vi "Setup.vi"(8 "error in (no error)":errorcluster caption="Fehler (Eingang, kein Fehler)", 9 "Baudrate":u32=250000, 10 "VISA resource name":refnum<visa-resource-name>, 11 "MoveoSerial Eingang":refnum<class "MoveoSerial.lvclass">) -> (0 "error out":errorcluster caption="Fehler (Ausgang)", 3 "MoveoSerial Ausgang":refnum<class "MoveoSerial.lvclass">)   [LabVIEW 2019, in "MoveoSerial.lvclass"]
uses:
  MoveoSerial.lvclass
  MoveoSerial.lvclass/MoveoSerial.ctl
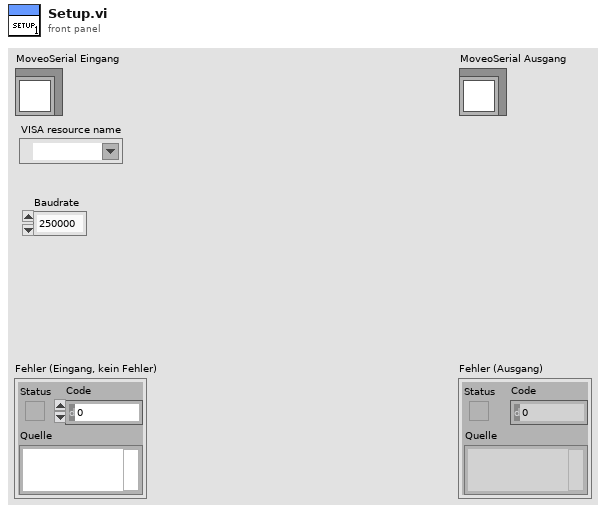
[diagram p1: front panel]
types:
  T1 = typedef "Serial - Settings.ctl" = cluster{"Baudrate":u32, "Datenbits":u16, "Parität":enum16{"None", "Odd", "Even", "Mark", "Space"}, "Stoppbits":u16, "Ablaufsteuerung":u16}
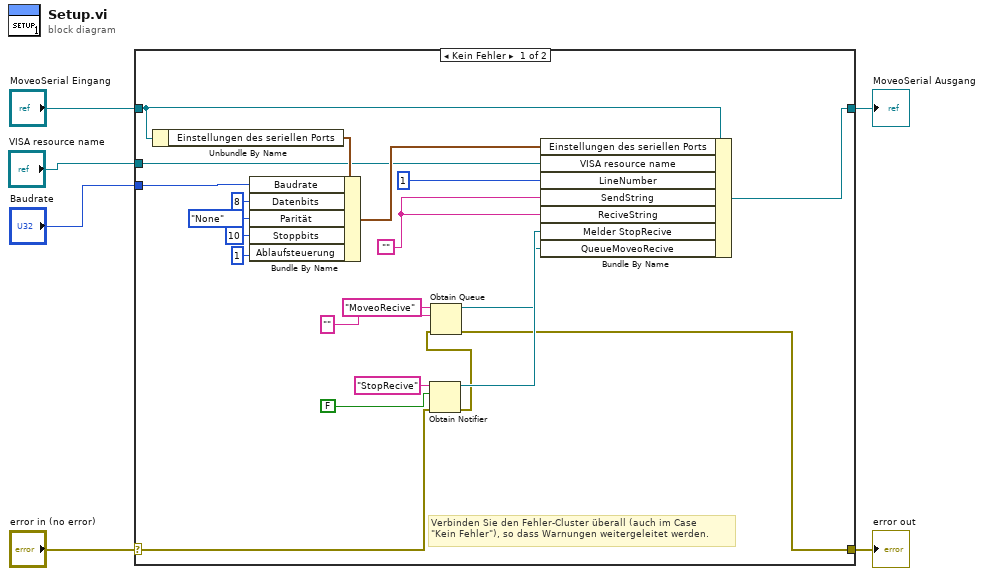
[diagram p0: block diagram]
diagram:
  n1 = case shown="Kein Fehler" "error in (no error)" {
    selector: "error in (no error)" -> [w13 w29]
    tunnel: [w10 w29] -> w5
    tunnel: [w27 w28] -> w3
    tunnel: "MoveoSerial Eingang" -> [w26 w28]
    tunnel: "Baudrate" -> [w19 _]
    tunnel: "VISA resource name" -> [w18 _]
    frame No Error {
      w16 = ""
      # "Verbinden Sie den Fehler-Cluster überall (auch im Case\n\"Kein Fehler\"), so dass Warnungen weitergeleitet werden."
      n2 = Unbundle By Name(w26) -> ("Einstellungen des seriellen Ports"=w25:T1)
      n3 = Bundle By Name(cluster=w25, "Baudrate"=w19, "Datenbits"=u16 8, "Parität"=enum16{"None", "Odd", "Even", "Mark", "Space"}."None", "Stoppbits"=u16 10, "Ablaufsteuerung"=u16 1) -> (w24:T1)
      n4 = Obtain Notifier(name (unnamed)="StopRecive" ("Name (unbenannt)"), notification data type=FALSE, error in (no error)=w13) -> (notifier out=w12:refnum<notifier>, error out=w11:errorcluster)  [unwired: 1 in, 1 out]
      n5 = Obtain Queue(name (unnamed)="MoveoRecive" ("Name (unbenannt)"), element data type="", error in (no error)=w11) -> (queue out=w9:refnum<queue>, error out=w10:errorcluster)  [unwired: 2 in, 1 out]
      n6 = Bundle By Name(cluster=w26, "Einstellungen des seriellen Ports"=w24, "VISA resource name"=w18, "LineNumber"=u64 1, "SendString"=w16, "ReciveString"=w16, "Melder StopRecive"=w12, "QueueMoveoRecive"=w9) -> (w27:refnum<class "MoveoSerial.lvclass">)
    }
    frame Error {
    }
  }
  "error out" <- w5
  "MoveoSerial Ausgang" <- w3
